vi "GetClassAttributes.vi"(5 "error in (no error)":errorcluster) -> (12 "created new":bool, 15 "ClassAttr":i32, 19 "error out":errorcluster)   [LabVIEW 2017, in "G#BaseClass2.lvclass"]
uses:
  G#BaseClass2.lvclass
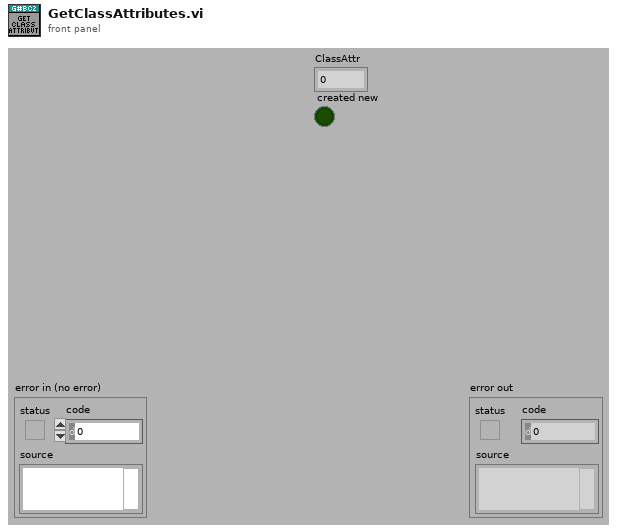
[diagram p1: front panel]
types:
  T1 = typedef "G#BaseClass2.lvclass/ClassAttributes.ctl" = cluster{"ClassAttr":i32}
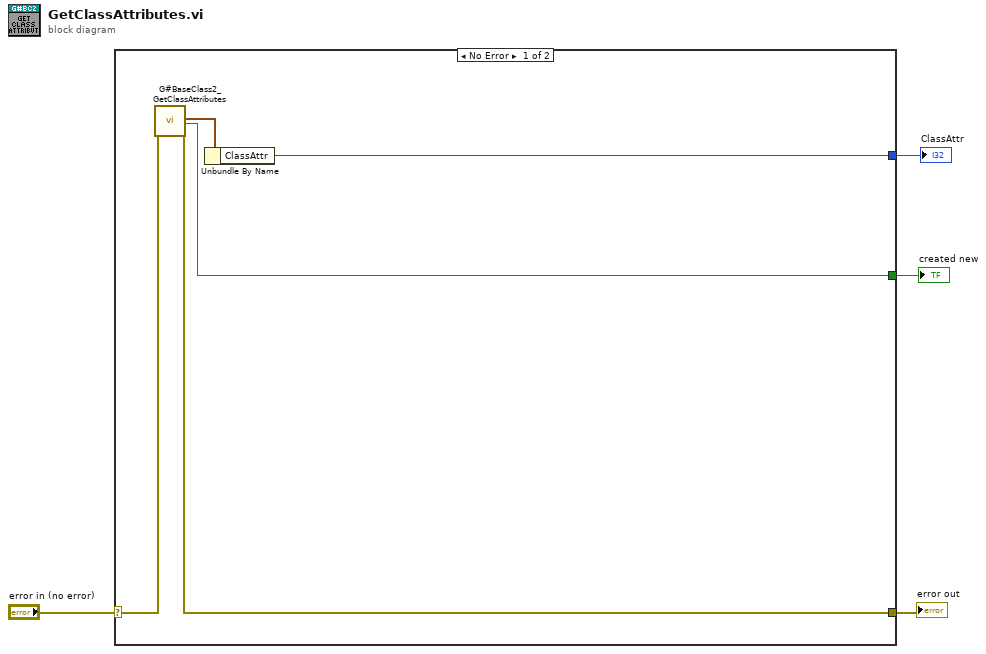
[diagram p0: block diagram]
diagram:
  n1 = case shown="No Error" "error in (no error)" {
    selector: "error in (no error)" -> [w9 w10]
    tunnel: [w8 w10] -> w3
    tunnel: [w6 _] -> w2
    tunnel: [w5 _] -> w1
    frame No Error {
      n2 = call "G#BaseClass2_GetClassAttributes.vi"("error in (no error)"=w9) -> ("class attributes"=w7:T1, "created new"=w5:bool, "error out"=w8:errorcluster)  [unwired: 14 in, 2 out]
      n3 = Unbundle By Name(w7) -> ("ClassAttr"=w6:i32)
    }
    frame Error {
    }
  }
  "error out" <- w3
  "ClassAttr" <- w2
  "created new" <- w1
